vi "개별읽기(Main).vi"() -> ()   [LabVIEW 2014]
panel:
  out "Word 배열(U16)":u16[](array[numeric])=[4096, 24576, 0, 0] format="%.0x"
  in  "직접변수":string[](array[string])=["%DW0000", "%DW0005", "%DW0010", "%PW000"]
  out "에러 출력":errorcluster
  in  "주소":string="192.168.0.10"
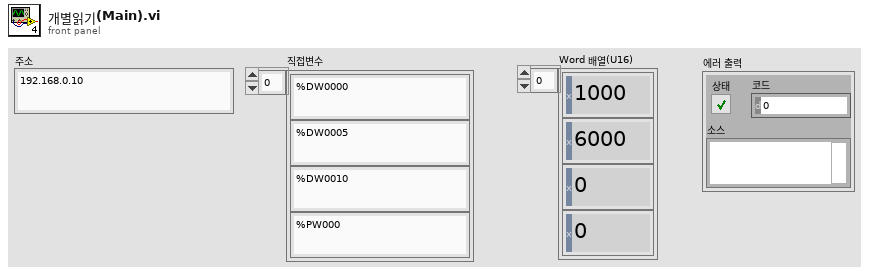
[diagram p1: front panel]
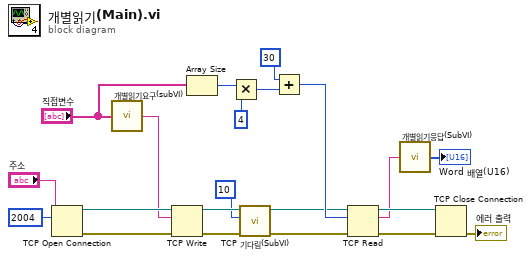
[diagram p0: block diagram]
diagram:
  n1 = TCP Open Connection(address="주소", remote port or service name=u16 2004 ("원격 포트 또는 서비스 이름")) -> (connection ID=w19:refnum<k5>, error out=w18:errorcluster)  [unwired: 3 in]
  n2 = call "개별읽기요구(subVI).vi"("직접변수"="직접변수") -> ("개별읽기"=w14:string)
  n3 = TCP Write(connection ID=w19, data in=w14, error in (no error)=w18) -> (connection ID out=w5:refnum<k5>, error out=w3:errorcluster)  [unwired: 1 in, 1 out]
  n4 = Array Size(array="직접변수") -> (size(s)=w12:i32)
  n5 = Multiply(x=w12, y=4) -> (x*y=w10:i32)
  n6 = call "TCP 기다림(SubVI).vi"("error in"=w3, "기다림(ms)"=u32 10, "TCP 네트워크 연결 입력"=w5) -> ("error out"=w2:errorcluster, "TCP 네트워크 연결 출력"=w4:refnum<k5>)  [unwired: 7 in]
  n7 = Add(x=30, y=w10) -> (x+y=w8:i32)
  n8 = TCP Read(connection ID=w4, bytes to read=w8, error in (no error)=w2) -> (connection ID out=w17:refnum<k5>, data out=w7:string, error out=w16:errorcluster)  [unwired: 2 in]
  n9 = call "개별읽기응답(SubVI).vi"("응답 프레임"=w7) -> ("Word 배열(U16)"=→"Word 배열(U16)":u16[])
  n10 = TCP Close Connection(connection ID=w17, error in (no error)=w16) -> (error out=→"에러 출력":errorcluster)  [unwired: 1 in, 1 out]
